vi "Choreo_Choreo_DifferentialLTVController.vi"(8 "Auto":bool=TRUE, 10 "ChoreoDifferentialSample":T6={"timestamp"=-999.0, "x"=0.0, "y"=0.0, "heading"=0.0, "velocityL"=0.0, "velocityR"=0.0, "angularVelocity"=0.0, "accelL"=0.0, "accelR"=0.0, "accelAngular"=0.0, "forceL"=0.0, "forceR"=0.0}, 11 "Current Position":T3={"TRANSLATION"={"X"=0.0, "Y"=0.0}, "ROTATION"={"VALUE"=0.0, "COS"=1.0, "SIN"=0.0}} {"ROTATION"."SIN" format="%13.4f"; "ROTATION"."COS" format="%13.4f"; "ROTATION"."VALUE" format="%13.4f"; "TRANSLATION"."Y" format="%14.3f"; "TRANSLATION"."X" format="%14.3f"}) -> (2 "On Target":bool, 3 "Chassis Speed Dmd":T2 {"vOmega" format="%10.3f"; "vY" format="%10.3f"; "vX" format="%10.3f"}, 4 "Ctrl Info":T1)   [LabVIEW 2019, in "ChoreoLib.lvlib"]
doc: "Creates and executes a differential drive control function to execute a Choreo Trajectory sample. The controller LTV controller.\n\nInputs:\n - Current Pose - pose2d - Current robot position pose calcualted by either Odometry or Pose Estimation.\n - ChoreoTrajectoryState - cluster - Trajectory state to execute\n - Auto - boolean - When TRUE closed loop control is used to control trajectory execution. This is mostly for debugging and robot tuning. (Optional. Default: TRUE )\n\nOutputs:\n - Choreo Speed Demand - chassis speed - Desired chassis speed (M/S, Rad/Sec)\n - On Target - boolean - TRUE when robot position is within tolerance of trajectory position\n - Ctrl Info - cluster - Information on control. Mostly for diagnostics."
uses:
  ChoreoLib.lvlib
  TypeDef/ChoreoDifferentialSample.ctl
  <vilib>/Rock Robotics/WPI/ThirdParty/JAS_Junk/TrajLib/TypeDef/POSE2D.ctl
  <vilib>/Rock Robotics/WPI/ThirdParty/JAS_Junk/TrajLib/TypeDef/TRANSLATION2D.ctl
  <vilib>/Rock Robotics/WPI/ThirdParty/JAS_Junk/TrajLib/TypeDef/ROTATION2D.ctl
  <vilib>/Rock Robotics/WPI/ThirdParty/JAS_Junk/TrajLib/TypeDef/CHASSIS_SPEEDS.ctl
  <vilib>/Rock Robotics/WPI/ThirdParty/JAS_Junk/TrajLib/ChassisSpeeds_New.vi
  <vilib>/Rock Robotics/WPI/ThirdParty/JAS_Junk/TrajLib/Pose2d_New.vi
  <vilib>/Rock Robotics/WPI/ThirdParty/JAS_Junk/TrajLib/Rotation2d_CreateAngle.vi
  <vilib>/Rock Robotics/WPI/ThirdParty/JAS_Junk/TrajLib/Translation2d_Create.vi
  <vilib>/Rock Robotics/WPI/ThirdParty/JAS_Junk/TrajLib/Trajectory_Library.lvlib
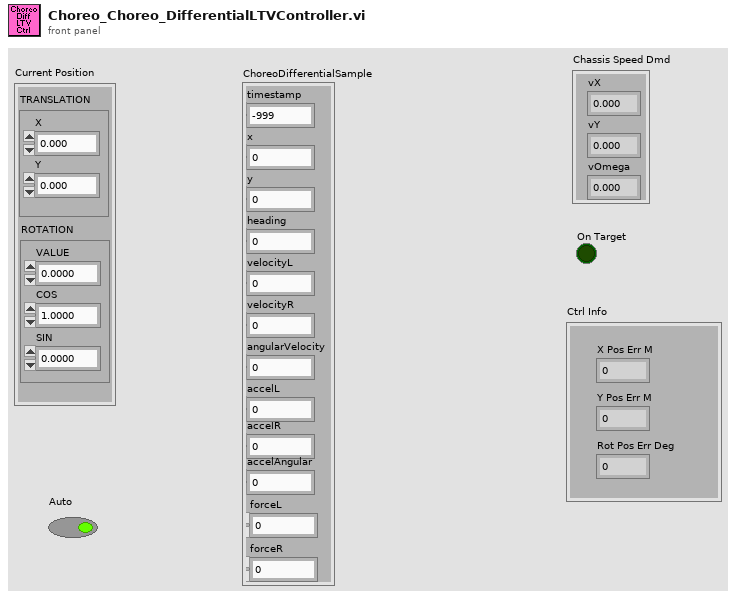
[diagram p1: front panel]
types:
  T1 = cluster{"X Pos Err M":dbl, "Y Pos Err M":dbl, "Rot Pos Err Deg":dbl}
  T2 = typedef "Trajectory_Library.lvlib/CHASSIS_SPEEDS.ctl" = cluster{"vX":dbl, "vY":dbl, "vOmega":dbl}
  T3 = typedef "Trajectory_Library.lvlib/POSE2D.ctl" = cluster{"TRANSLATION":T4, "ROTATION":T5}
  T4 = typedef "Trajectory_Library.lvlib/TRANSLATION2D.ctl" = cluster{"X":dbl, "Y":dbl}
  T5 = typedef "Trajectory_Library.lvlib/ROTATION2D.ctl" = cluster{"VALUE":dbl, "COS":dbl, "SIN":dbl}
  T6 = typedef "ChoreoLib.lvlib/ChoreoDifferentialSample.ctl" = cluster{"timestamp":dbl, "x":dbl, "y":dbl, "heading":dbl, "velocityL":dbl, "velocityR":dbl, "angularVelocity":dbl, "accelL":dbl, "accelR":dbl, "accelAngular":dbl, "forceL":dbl, "forceR":dbl}
  T7 = typedef "Trajectory_Library.lvlib/LTV_UNICYCLE_CONTROLLER_MODEL_PARAMS.CTL" = cluster{"Max linear ctrl effort M/S":dbl, "Max angular ctrl effort Rad/S":dbl, "Max Heading Meas Tol Rad":dbl, "Max X Pos Meas Tol M":dbl, "Max Y Pos Meas Tol M":dbl, "Max Linear Vel M/S":dbl}
  T8 = typedef "Trajectory_Library.lvlib/LTV_UNICYCLE_CONTROLLER_TOLERANCE.CTL" = cluster{"Max Heading Tolerance Rad":dbl, "Max X Tolerance M":dbl, "Max Y Tolerance M":dbl}
  T9 = typedef "Trajectory_Library.lvlib/LTV_UNICYCLE_CONTROLLER.ctl" = cluster{"States":i32, "Inputs":i32, "PoseError":T3, "PoseTolerance":T3, "Dt":dbl, "Enabled":bool, "LQR_K_Table":T10}
  T10 = typedef "Trajectory_Library.lvlib/FUNCTION_GENERATOR_MATRIX.ctl" = cluster{"Table Xs":dbl[], "Table Ys":variant[], "MinX":dbl, "MaxX":dbl, "ItemCount":i32, "Rows":i32, "Columns":i32}
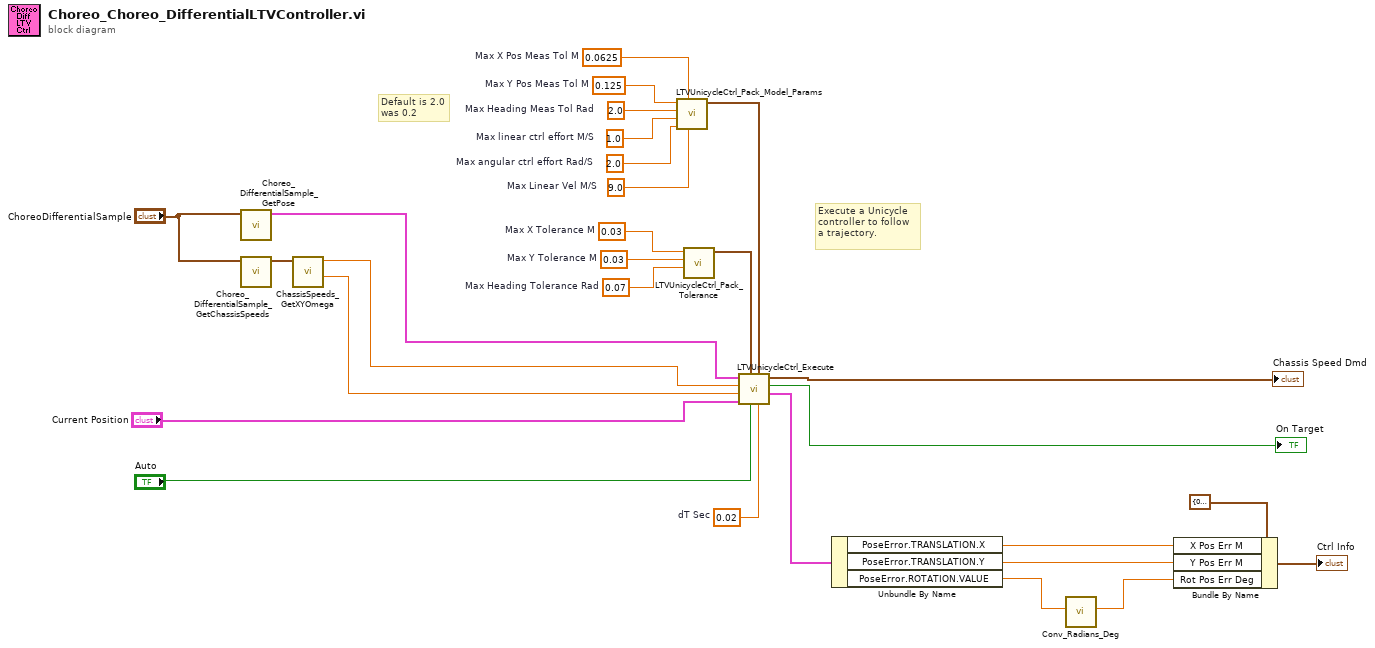
[diagram p0: block diagram]
diagram:
  w9 = 0.02  # dT Sec
  w17 = 0.03  # Max X Tolerance M
  w18 = 0.03  # Max Y Tolerance M
  w19 = 0.07  # Max Heading Tolerance Rad
  w20 = 0.125  # Max Y Pos Meas Tol M
  w21 = 2.0  # Max Heading Meas Tol Rad
  w22 = 1.0  # Max linear ctrl effort M/S
  w23 = 2.0  # Max angular ctrl effort Rad/S
  w24 = 0.0625  # Max X Pos Meas Tol M
  w25 = 9.0  # Max Linear Vel M/S
  # "Default is 2.0\nwas 0.2"
  # "Execute a Unicycle\ncontroller to follow\na trajectory."
  n1 = call "Choreo_DifferentialSample_GetPose.vi"("ChoreoDifferentialSample"="ChoreoDifferentialSample") -> ("Pose"=w16:T3)  [unwired: 10 in]
  n2 = call "Choreo_DifferentialSample_GetChassisSpeeds.vi"("ChoreoDifferentialSample"="ChoreoDifferentialSample") -> ("ChassisSpeeds"=w14:T2)  [unwired: 10 in]
  n3 = call <vilib>:"ChassisSpeeds_GetXYOmega.vi"("CHASSIS"=w14) -> ("vAngular"=w12:dbl, "vX"=w13:dbl)  [unwired: 8 in, 1 out]
  n4 = call <vilib>:"LTVUnicycleCtrl_Pack_Model_Params.vi"("Max Linear Vel M/S"=w25, "Max X Pos Meas Tol M"=w24, "Max angular ctrl effort Rad/S"=w23, "Max linear ctrl effort M/S"=w22, "Max Heading Meas Tol Rad"=w21, "Max Y Pos Meas Tol M"=w20) -> ("LTV_Unicycle_Ctrl_Model _Params"=w26:T7)  [unwired: 5 in]
  n5 = call <vilib>:"LTVUnicycleCtrl_Pack_Tolerance.vi"("Max Heading Tolerance Rad"=w19, "Max Y Tolerance M"=w18, "Max X Tolerance M"=w17) -> ("LTV_Unicycle_Ctrl_Tolerance"=w27:T8)  [unwired: 8 in]
  n6 = call <vilib>:"LTVUnicycleCtrl_Execute.vi"("dT Sec"=w9, "LTV_Unicycle_Ctrl_Model"=w26, "Enabled"="Auto", "LTV_Unicycle_Ctrl_Tolerance"=w27, "CurrentPose"="Current Position", "RefAngularVelocity"=w12, "RefLinearVelocity"=w13, "RefPose"=w16) -> ("out LTV_UNICYCLE_CONTROLLER"=w6:T9, "At Reference"=→"On Target":bool, "ChassisSpeeds"=→"Chassis Speed Dmd":T2)  [unwired: 1 out]
  n7 = Unbundle By Name(w6) -> ("PoseError.TRANSLATION.X"=w5:dbl, "PoseError.TRANSLATION.Y"=w4:dbl, "PoseError.ROTATION.VALUE"=w3:dbl)
  n8 = call <vilib>:"Conv_Radians_Deg.vi"("Radians"=w3) -> ("Degrees"=w28:dbl)  [unwired: 10 in]
  n9 = Bundle By Name(cluster=T1 {"X Pos Err M"=0.0, "Y Pos Err M"=0.0, "Rot Pos Err Deg"=0.0} ("Ctrl Info"), "X Pos Err M"=w5, "Y Pos Err M"=w4, "Rot Pos Err Deg"=w28) -> (→"Ctrl Info":T1)
